vi "2 - Termômetro.vi"() -> ()   [LabVIEW 2020]
uses:
  1962017e-d4fb-4c6c-8f52-68fff2feb30f.vi
panel:
  out "Histórico (Term. 1)":dbl(graph)
  out "Termômetro 2":dbl(slide) scale=-50.0..250.0
  in  "Conversão":bool
  out "Termômetro 1":dbl(slide) scale=0.0..100.0
  in  "Temperatura":dbl(knob) scale=0.0..100.0
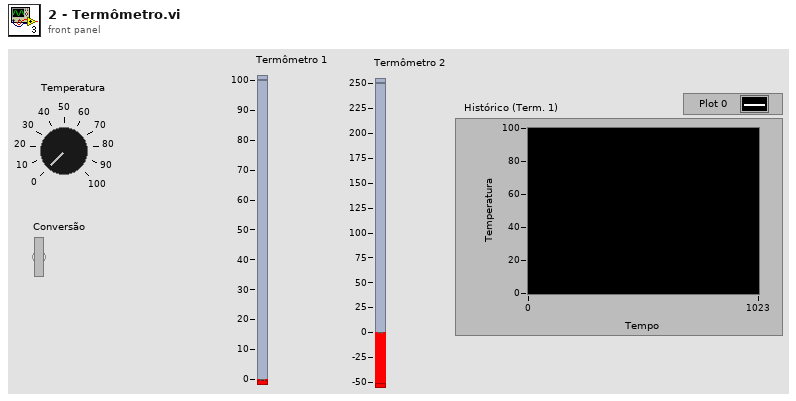
[diagram p1: front panel]
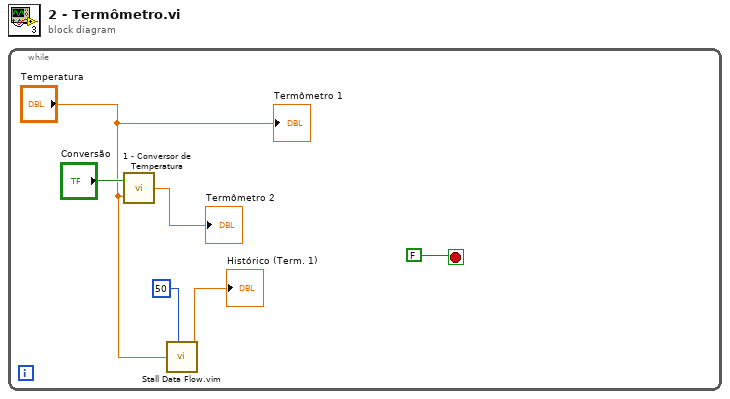
[diagram p0: block diagram]
diagram:
  n1 = while {
    stop <- FALSE stop-if-true
    n2 = call "1 - Conversor de Temperatura.vi"("Entrada"="Temperatura", "(F) C -> F\n(T) F -> C"="Conversão") -> ("Saída"=→"Termômetro 2":dbl)
    n3 = call "Stall Data Flow.vim"("value in"="Temperatura", "milliseconds to wait"=50) -> ("value out"=→"Histórico (Term. 1)":dbl)  [unwired: 1 out]
    "Termômetro 1" <- "Temperatura"
  }
